vi "Operator Login Dialog.vi"(8 "error in (no error)":errorcluster, 9 "contextType":i32(ring) items=["Machine", "Domain", "ApplicationDirectory"], 11 "Company Name":string) -> (0 "error out":errorcluster, 1 "Groups":string[](array[string]), 2 "Operator Name":string, 3 "Logged In?":bool)   [LabVIEW 2020, in "Login Dialogs.lvlib"]
doc: "This Dialog Box will authenticate the user based on its local windows account"
uses:
  Login Dialogs.lvlib
  System.DirectoryServices.AccountManagement
panel:
  in  "Password":string
  in  "User Name":string
  in  "Cancel":bool
  in  "Login":bool
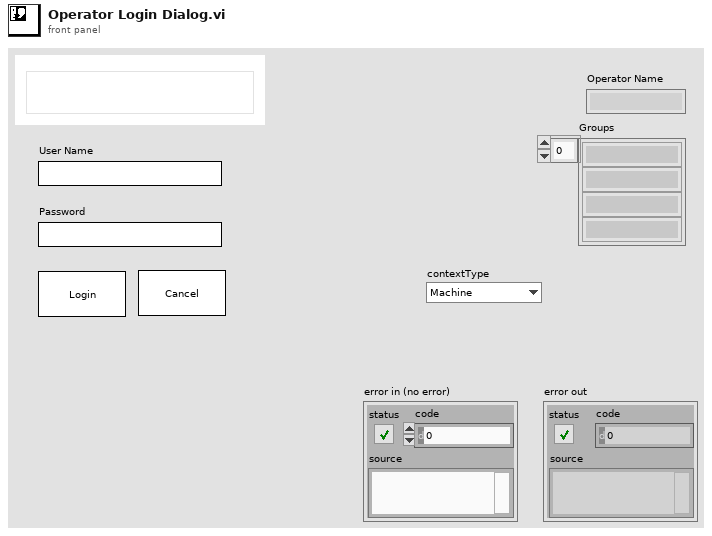
[diagram p1: front panel]
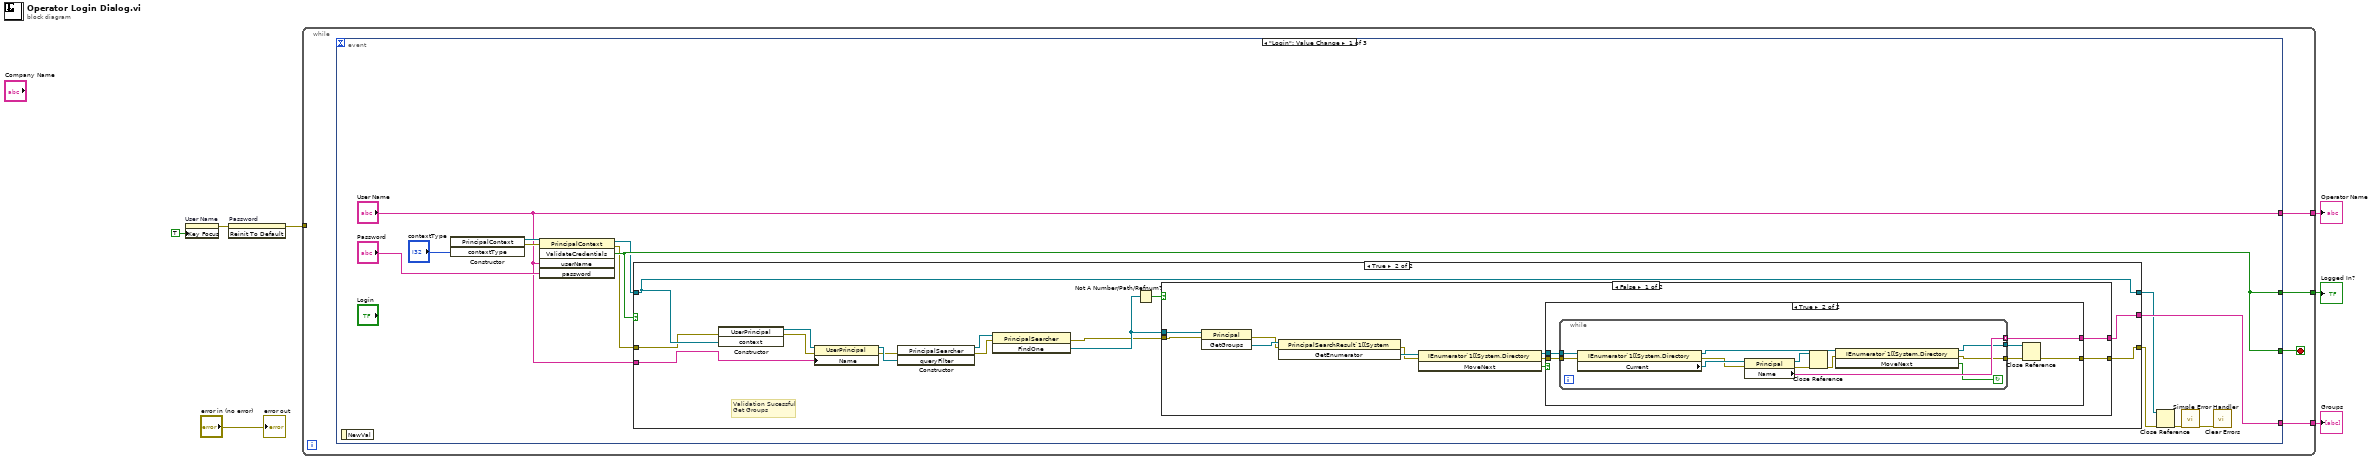
[diagram p0: block diagram]
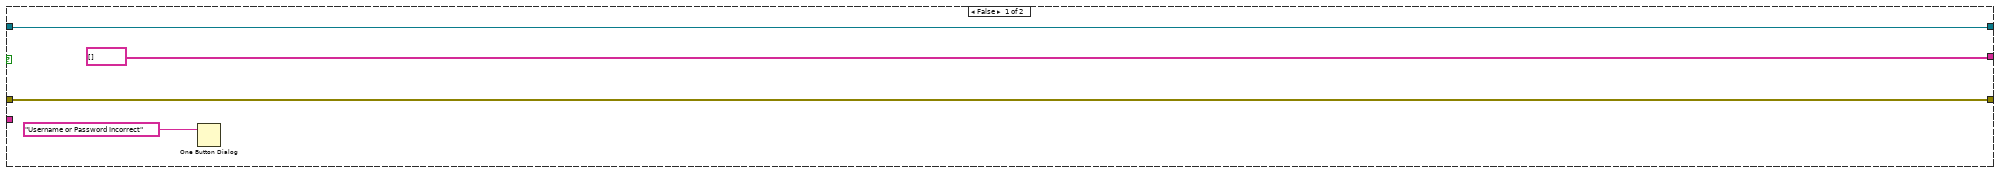
[diagram p2: hidden frame]
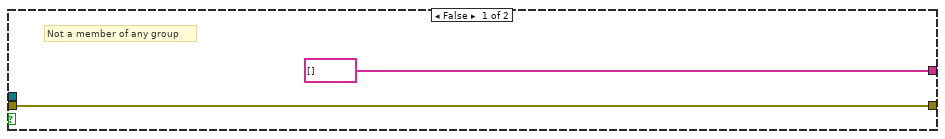
[diagram p3: hidden frame]
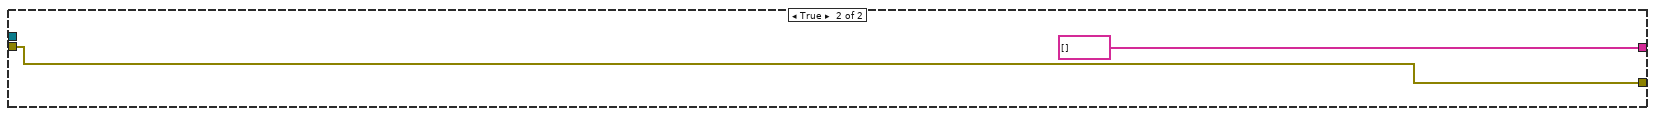
[diagram p4: hidden frame]
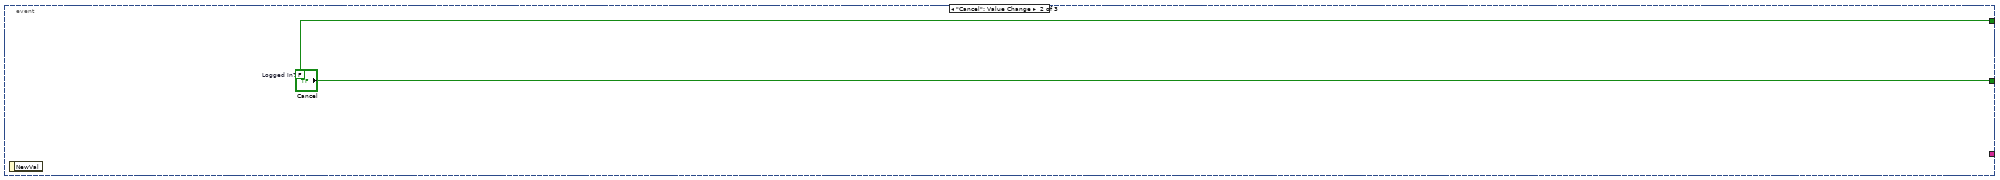
[diagram p5: hidden frame]
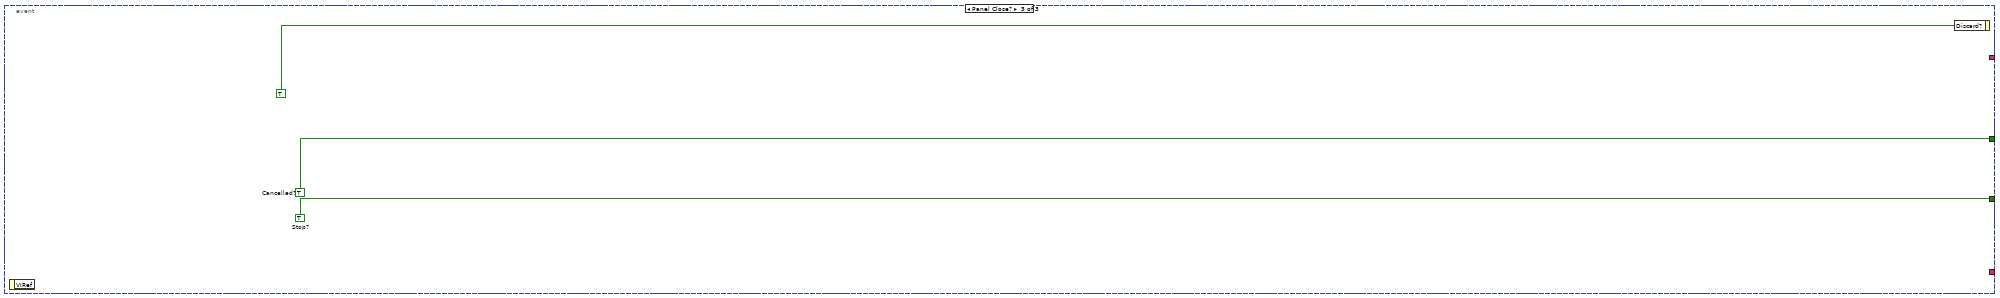
[diagram p6: hidden frame]
diagram:
  n1 = property on="User Name" class="Str"("Key Focus"=TRUE) -> (error out=w1:errorcluster)  [unwired: 2 in, 1 out]
  n2 = invoke on="Password" class="Str" method="Reinit To Default"(error in=w1) -> (error out=w4:errorcluster)  [unwired: 2 in, 2 out]
  n3 = while {
    tunnel: [w10] -> w7
    tunnel: [w9] -> w6
    tunnel: [w8] -> w5
    tunnel: w4 -> [_]
    stop <- w11 stop-if-true
    n4 = event shown="[0] \"Login\": Value Change" {
      selector: _ -> [_ _ _]
      dyn-events: _ -> [_ _ _]
      timeout: _ -> [_ _ _]
      tunnel: [w20 "Cancel" w79] -> w11
      tunnel: [w20 w77 w78] -> w10
      tunnel: ["User Name" _ _] -> w9
      tunnel: [w17 _ _] -> w8
      event "Login": Value Change {
        n5 = event-data() -> ()  [unwired: 1 in, 1 out]
        n6 = constructor class="PrincipalContext"("contextType"="contextType") -> (reference out=w22:refnum<k24>, error out=w23:errorcluster)  [unwired: 3 in, 2 out]
        n7 = invoke class="PrincipalContext" method="ValidateCredentials"(reference=w22, error in=w23, "userName"="User Name", "password"="Password") -> (reference out=w16:refnum<k24>, error out=w15:errorcluster, "ValidateCredentials"=w20:bool)  [unwired: 1 in, 2 out]
        n8 = case shown="True" w20 {
          tunnel: [string[] [] ("Groups") w38] -> w17
          tunnel: w16 -> [w26 w42]
          tunnel: w15 -> [w27 w35]
          tunnel: [w27 w37] -> w14
          tunnel: [w26 w42] -> w13
          tunnel: "User Name" -> [_ w41]
          frame False {
            n9 = One Button Dialog(message="Username or Password Incorrect") -> ()  [unwired: 1 in, 1 out]
          }
          frame True {
            # "Validation Sucessful\nGet Groups"
            n10 = constructor class="UserPrincipal"(error in=w35, "context"=w42) -> (reference out=w34:refnum<k24>, error out=w33:errorcluster)  [unwired: 2 in, 2 out]
            n11 = property class="UserPrincipal"(reference=w34, error in=w33, "Name"=w41) -> (reference out=w32:refnum<k24>, error out=w31:errorcluster)
            n12 = constructor class="PrincipalSearcher"(error in=w31, "queryFilter"=w32) -> (reference out=w29:refnum<k24>, error out=w30:errorcluster)  [unwired: 2 in, 2 out]
            n13 = invoke class="PrincipalSearcher" method="FindOne"(reference=w29, error in=w30) -> (error out=w36:errorcluster, "FindOne"=w40:refnum<k24>)  [unwired: 1 in, 1 out]
            n14 = Not A Number/Path/Refnum?(number/path/refnum=w40) -> (NaN/Path/Refnum?=w39:bool)
            n15 = case shown="False" w39 {
              tunnel: w40 -> [w53 _]
              tunnel: [w47 string[] [] ("Groups")] -> w38
              tunnel: [w45 w75] -> w37
              tunnel: w36 -> [w44 w75]
              frame False {
                n16 = invoke class="Principal" method="GetGroups"(reference=w53, error in=w44) -> (error out=w43:errorcluster, "rvices.AccountManagement, Version=0.0.0.0, Culture=neutral, PublicKeyToken=b77a5c561934e089\tGetGroups"=w52:refnum<k24>)  [unwired: 1 in, 1 out]
                n17 = invoke class="PrincipalSearchResult`1[[System" method="GetEnumerator"(reference=w52, error in=w43) -> (error out=w50:errorcluster, "GetEnumerator"=w51:refnum<k24>)  [unwired: 1 in, 1 out]
                n18 = invoke class="IEnumerator`1[[System.Directory" method="MoveNext"(reference=w51, error in=w50) -> (reference out=w49:refnum<k24>, error out=w46:errorcluster, "MoveNext"=w48:bool)  [unwired: 1 in]
                n19 = case shown="True" w48 {
                  tunnel: w49 -> [_ w61]
                  tunnel: [string[] [] ("Groups") w59] -> w47
                  tunnel: w46 -> [w54 w60]
                  tunnel: [w54 w56] -> w45
                  frame False {
                    # "Not a member of any group"
                  }
                  frame True {
                    n20 = while {
                      tunnel: w61 -> [w73]
                      tunnel: w60 -> [w72]
                      tunnel: [w68] -> w59 mode=indexing
                      tunnel: [w66] -> w58
                      tunnel: [w62] -> w57
                      stop <- w67 continue-if-true
                      n21 = property class="IEnumerator`1[[System.Directory"(reference=w73, error in=w72) -> (reference out=w69:refnum<k24>, error out=w70:errorcluster, "Current"=w71:refnum<k24>)
                      n22 = property class="Principal"(reference=w71, error in=w70) -> (reference out=w65:refnum<k24>, error out=w64:errorcluster, "Name"=w68:string)
                      n23 = Close Reference(reference=w65, error in (no error)=w64) -> (error out=w63:errorcluster)
                      n24 = invoke class="IEnumerator`1[[System.Directory" method="MoveNext"(reference=w69, error in=w63) -> (reference out=w62:refnum<k24>, error out=w66:errorcluster, "MoveNext"=w67:bool)  [unwired: 1 in]
                    }
                    n25 = Close Reference(reference=w57, error in (no error)=w58) -> (error out=w56:errorcluster)
                  }
                }
              }
              frame True {
              }
            }
          }
        }
        n26 = Close Reference(reference=w13, error in (no error)=w14) -> (error out=w19:errorcluster)
        n27 = call <vilib>:"Simple Error Handler.vi"("error in (no error)"=w19) -> ("error out"=w18:errorcluster)  [unwired: 4 in, 4 out]
        n28 = call <vilib>:"Clear Errors.vi"("error in (no error)"=w18) -> ()  [unwired: 5 in, 2 out]
      }
      event "Cancel": Value Change {
        w77 = FALSE  # Logged In?
        n29 = event-data() -> ()  [unwired: 1 in, 1 out]
      }
      event Panel Close? {
        w78 = TRUE  # Cancelled?
        w79 = TRUE  # Stop?
        n30 = event-data() -> ()  [unwired: 1 in, 1 out]
        n31 = event-data("Discard?"=TRUE) -> ()  [unwired: 1 in, 1 out]
      }
    }
  }
  "Logged In?" <- w7
  "Operator Name" <- w6
  "Groups" <- w5
  "error out" <- "error in (no error)"
